vi "1-Tap 8-bit Camera with Bayer (Host).vi"() -> ()   [LabVIEW 2012]
doc: "This is the host VI for the 1-Tap 8-Bit Camera with Bayer example. This example demonstrates how to acquire images from a 1-tap, 8-bit, base configuration, Camera Link camera with a color sensor and display the images on the host.\n\nThis example also demonstrates the use of third-party IP imported into the LabVIEW project as a CLIP. In this case, the imported CLIP comes from an FPGA netlist and performs the Bayer color decoding to convert the incoming 8-bit Bayer images into 24-bit RGB images in real time.\n\nAdditionally, the example demonstrates the serial server, which allows third-party camera configuration utilities to communicate with the camera using the Camera Link serial interface while this VI is running."
uses:
  <vilib>/userdefined/High Color/nirio_resource_hc.ctl
  <vilib>/FPGAPlugInAG/PCIe-1473R/niLvFpga_Open_PCIe-1473R.vi
  <vilib>/rvi/interface/common/dynamic/niFpgaDynamicAddResources.vi
  <vilib>/FPGAPlugInAG/Dynamic/niLvFpga_Reset_Dynamic.vi
  <vilib>/Utility/error.llb/Error Cluster From Error Code.vi
  <vilib>/rvi/errors/niLvFpgaAdjustHostInterfaceError.vi
  <vilib>/FPGAPlugInAG/Dynamic/niLvFpga_Run_Dynamic.vi
  <vilib>/FPGAPlugInAG/Dynamic/niLvFpga_Close_Dynamic.vi
  <vilib>/rvi/interface/nirviOpenFPGA/nirviOpenFPGA.xnode
  FPGA Bitfiles/1-Tap8-bitCamera_FPGATarget_1-Tap8-bitCamera_6EA2B931.lvbitx
  1-Tap 8-Bit Camera with Bayer (FPGA).vi
  <vilib>/rvi/interface/nirviMethod/nirviMethod.xnode
  <vilib>/rvi/interface/nirviReadWriteControl/nirviReadWriteControl.xnode
  <vilib>/rvi/interface/nirviCloseFPGA/nirviCloseFPGA.xnode
  NiFpgaLv.dll
  <vilib>/rvi/interface/Simulation/niFpgaSimulationCallBeginRW.vi
  <vilib>/rvi/errors/niLvFpgaMergeErrorWithErrorCode.vi
  <vilib>/FPGAPlugInAG/Dynamic/niLvFpga_ConfigureFifo_Dynamic.vi
  <vilib>/FPGAPlugInAG/Dynamic/niLvFpga_StartFifo_Dynamic.vi
  <vilib>/FPGAPlugInAG/Dynamic/niLvFpga_ReadFifo_Dynamic.vi
panel:
  in  "Bayer Pattern":u16(ring) items=["GBGB::RGRG", "GRGR::BGBG", "BGBG::GRGR", "RGRG::GBGB"]
  out "Acq In Progress":bool
  in  "Frames To Acquire":u32=1 caption="Frames To Acquire\n(0 = infinite)"
  in  "Cancel":bool
  out "Acq'd Frame Width":u32
  in  "Stopped":bool
  in  "RIO Device":T1="RIO0"
  out "DMA Write Timeout":bool
  in  "Start Serial Server":bool=TRUE
  out "Frames Acq'd":u32
  out "Acq'd Frame Height":u32
  out "Image":T2(plugin-control)
  in  "Acquire":bool
  in  "Stop":bool
  in  "Image Height":u32=480 max=65535
  in  "Image Width":u32=640 max=65535
  out "Initialized":bool
  # "Note: The decoded output image is two columns\nand two rows smaller than the input image."
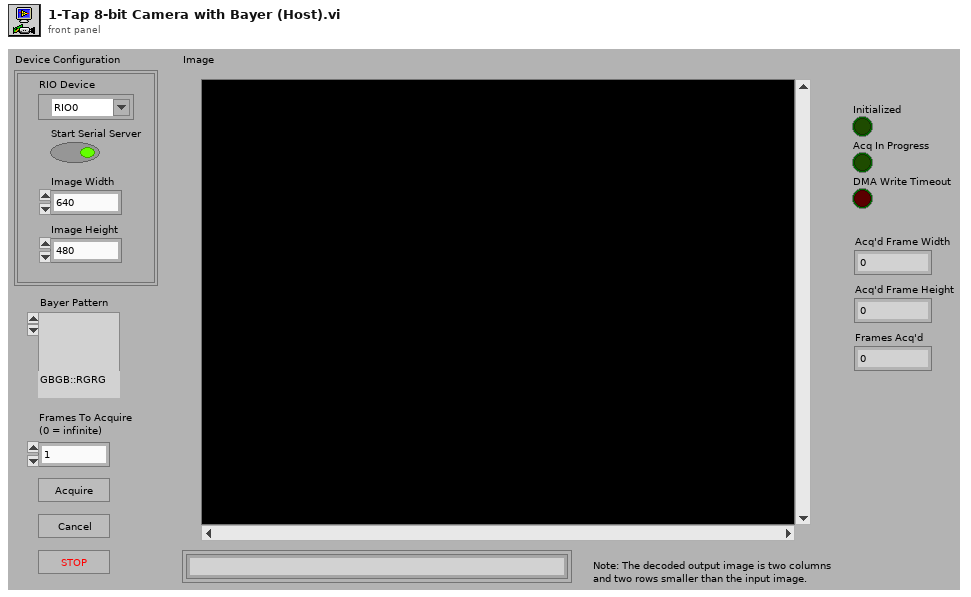
[diagram p1: front panel]
types:
  T1 = typedef "nirio_resource_hc.ctl" = tag
  T2 = typedef "IMAQ Image.ctl" = refnum<image>
  T3 = enum8{"Standard", "Basler 10-tap", "Vosskühler 10-tap"}
  T4 = typedef "Image Type" = u32
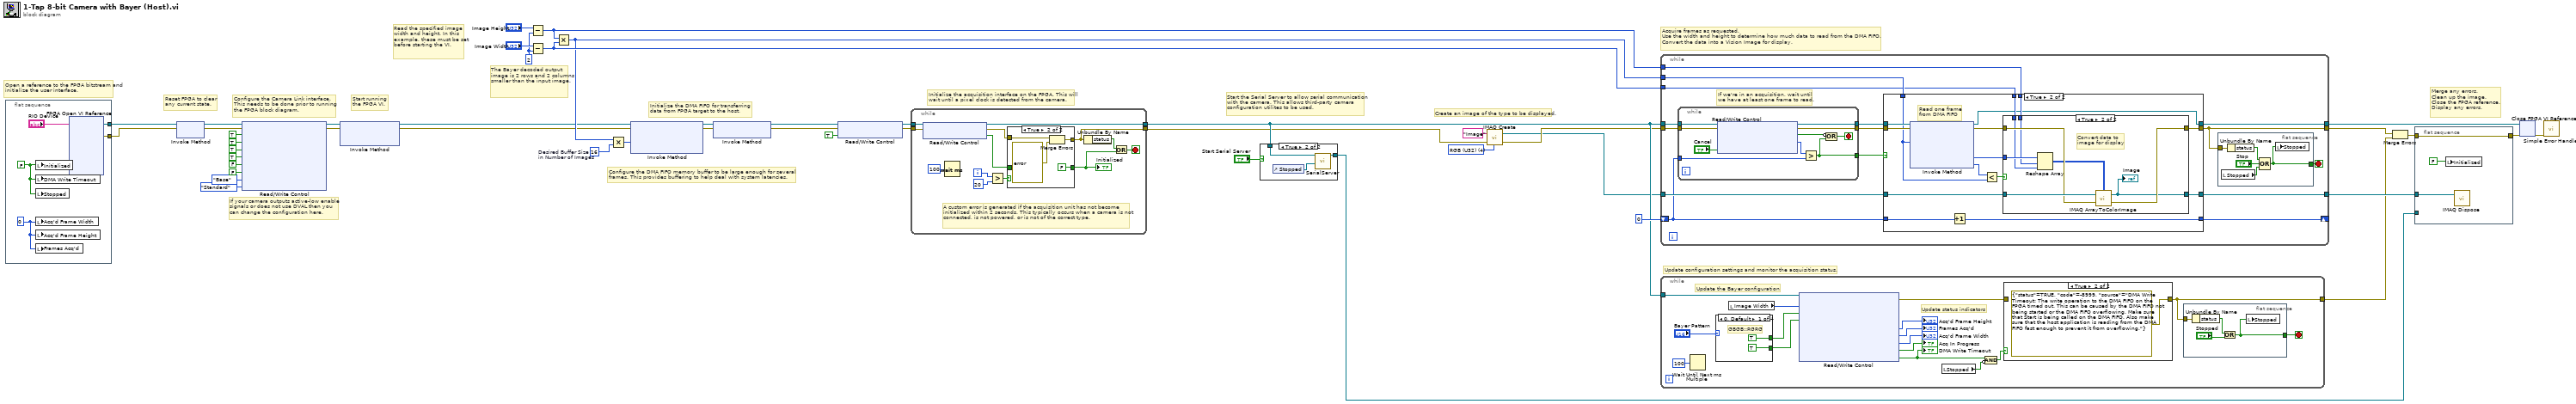
[diagram p0: block diagram]
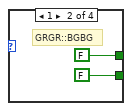
[diagram p3: hidden frame]
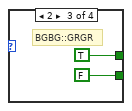
[diagram p4: hidden frame]
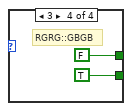
[diagram p5: hidden frame]
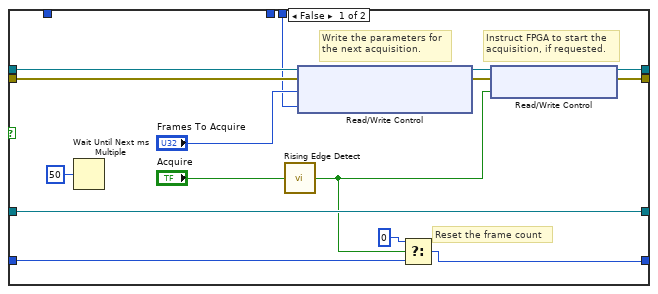
[diagram p7: hidden frame]
diagram:
  w6 = u32 2 ("y")
  w43 = T4 4 items=["Grayscale (U8)", "Grayscale (I16)", "Grayscale (SGL)", "Complex (CSG)", "RGB (U32)", "HSL (U32)", "RGB (U64)", "Grayscale (U16)"] ("Image Type")
  w17 = u32 16  # Desired Buffer Size in Number of Images
  # "The Bayer decoded output image is 2 rows and 2 columns smaller than the input image."
  # "If your camera outputs active-low enable\nsignals or does not use DVAL then you\ncan change the configuration here."
  # "Configure the DMA FIFO memory buffer to be large enough for several\nframes. This provides buffering to help deal with system latencies."
  # "Start running\nthe FPGA VI."
  # "Reset FPGA to clear\nany current state."
  # "Read the specified image width and height. In this example, these must be set before starting the VI."
  # "Merge any errors.\nClean up the image.\nClose the FPGA reference.\nDisplay any errors."
  # "Acquire frames as requested.\nUse the width and height to determine how much data to read from the DMA FIFO.\nConvert the data into a Vision Image for display."
  # "Update configuration settings and monitor the acquisition status."
  # "Start the Serial Server to allow serial communication\nwith the camera. This allows third-party camera\nconfiguration utilites to be used."
  # "Create an image of the type to be displayed."
  # "Initialize the acquisition interface on the FPGA. This will\nwait until a pixel clock is detected from the camera."
  # "Initialize the DMA FIFO for transferring\ndata from FPGA target to the host."
  # "Configure the Camera Link interface.\nThis needs to be done prior to running\nthe FPGA block diagram."
  # "Open a reference to the FPGA bitstream and initialize the user interface."
  n1 = flat-sequence {
    tunnel: [w49] -> w36
    tunnel: [w48] -> w47
    frame #0 {
      w52 = u32 0 ("Num Lines Acq'd")
      w51 = FALSE ("stop")
      n2 = local write "Initialized"(w51) -> ()
      n3 = local write "DMA Write Timeout"(w51) -> ()
      n4 = local write "Stopped"(w51) -> ()
      n5 = local write "Acq'd Frame Width"(w52) -> ()
      n6 = local write "Acq'd Frame Height"(w52) -> ()
      n7 = local write "Frames Acq'd"(w52) -> ()
      n8 = xnode "FPGA Open VI Reference"("resource name"="RIO Device") -> ("FPGA VI Reference Out"=w49:refnum<k20>, "error out"=w48:errorcluster)  [unwired: 1 in]
    }
  }
  n9 = xnode "Invoke Method"("FPGA VI Reference In"=w36, "error in"=w47) -> ("FPGA VI Reference Out"=w25:refnum<k20>, "error out"=w28:errorcluster)
  n10 = xnode "Read/Write Control"("FPGA VI Reference In"=w25, "error in"=w28, "CL Config.FVAL Active High"=TRUE ("IO Module Config.CL FVAL Active High"), "CL Config.LVAL Active High"=TRUE ("IO Module Config.CL LVAL Active High"), "CL Config.DVAL Active High"=TRUE ("IO Module Config.CL DVAL Active High"), "CL Config.Spare Active High"=TRUE ("IO Module Config.CL Spare Active High"), "CL Config.Line Scan"=FALSE ("Line Scan"), "Acq Control.Ignore DVAL"=FALSE ("CL Config.Line Scan"), "CL Config.Configuration"=enum8{"Base", "Medium", "Full"}."Base", "CL Config.Signal Mapping"=T3."Standard") -> ("FPGA VI Reference Out"=w29:refnum<k20>, "error out"=w27:errorcluster)
  n11 = xnode "Invoke Method"("FPGA VI Reference In"=w29, "error in"=w27) -> ("FPGA VI Reference Out"=w2:refnum<k20>, "error out"=w1:errorcluster)  [unwired: 1 in]
  n12 = Subtract(x="Image Height", y=w6) -> (x-y=w8:u32)
  n13 = Subtract(x="Image Width", y=w6) -> (x-y=w7:u32)
  n14 = Multiply(x=w8, y=w7) -> (x*y=w5:u32)
  n15 = Multiply(x=w5, y=w17) -> (x*y=w19:u32)
  n16 = xnode "Invoke Method"("FPGA VI Reference In"=w2, "error in"=w1, "Requested Depth"=w19) -> ("FPGA VI Reference Out"=w35:refnum<k20>, "error out"=w34:errorcluster)  [unwired: 1 out]
  n17 = xnode "Invoke Method"("FPGA VI Reference In"=w35, "error in"=w34) -> ("FPGA VI Reference Out"=w20:refnum<k20>, "error out"=w33:errorcluster)
  n18 = xnode "Read/Write Control"("FPGA VI Reference In"=w20, "error in"=w33, "Acq Control.Initialize"=TRUE ("Arm Acquisition")) -> ("FPGA VI Reference Out"=w46:refnum<k20>, "error out"=w45:errorcluster)
  n19 = while {
    tunnel: w46 -> [w60]
    tunnel: w45 -> [w59]
    tunnel: [w58] -> w16
    tunnel: [w62] -> w15
    i -> [w54]
    stop <- w65 stop-if-true
    # "A custom error is generated if the acquisition unit has not become initialized within 2 seconds. This typically occurs when a camera is not connected, is not powered, or is not of the correct type."
    n20 = xnode "Read/Write Control"("FPGA VI Reference In"=w60, "error in"=w59) -> ("FPGA VI Reference Out"=w58:refnum<k20>, "error out"=w57:errorcluster, "Acq Status.Initialized"=w56:bool)
    n21 = Wait (ms)(milliseconds to wait=u32 100) -> ()  [unwired: 1 out]
    n22 = Greater?(x=w54, y=20) -> (0:w55:bool)
    n23 = case shown="True" w55 {
      tunnel: [w67 FALSE] -> w61
      tunnel: w56 -> [w67 _]
      tunnel: w57 -> [w66 w69]
      tunnel: [w66 w71] -> w62
      frame False {
      }
      frame True {
        n24 = Merge Errors(w69, errorcluster {"status"=TRUE, "code"=-8999, "source"="Acquisition Initialization: This error typically occurs when a camera is not properly connected, is not powered, or is not of the correct type."} ("error in")) -> (w71:errorcluster)
      }
    }
    "Initialized" <- w61
    n25 = Unbundle By Name(w62) -> ("status"=w64:bool)
    n26 = Or(x=w64, y=w61) -> (x .or. y?=w65:bool)
  }
  n27 = case shown="True" "Start Serial Server" {
    tunnel: [_ w72] -> w37
    tunnel: w16 -> [_ w73]
    frame False {
    }
    frame True {
      n28 = control-ref of="Stopped"() -> (w74:refnum<vi>)
      n29 = call "SerialServer.vi"("Stop Refnum"=w74, "FPGA VI Reference In"=w73) -> ("FPGA VI Reference Out"=w72:refnum<k20>)  [unwired: 5 in]
    }
  }
  n30 = call "IMAQ Create"("Image Name"="Image", "Image Type"=w43, "error in (no error)"=w15) -> ("New Image"=w11:T2, "error out"=w12:errorcluster)  [unwired: 2 in]
  n31 = while {
    tunnel: w16 -> [w81]
    tunnel: w12 -> [w80]
    tunnel: w5 -> [w89]
    tunnel: w8 -> [w88]
    tunnel: w7 -> [w87]
    tunnel: w11 -> [w86]
    tunnel: [w84] -> w31
    tunnel: [w85] -> w42
    tunnel: [w82] -> w39
    shift-right: [w76] -> _
    shift-left: u32 0 -> [w75]
    stop <- w83 stop-if-true
    # "If we're in an acquisition, wait until \nwe have at least one frame to read."
    n32 = while {
      tunnel: w81 -> [w96]
      tunnel: w80 -> [w95]
      tunnel: [w93] -> w79
      tunnel: [w94] -> w78
      tunnel: w75 -> [w99]
      tunnel: [w97] -> w77
      stop <- w98 stop-if-true
      n33 = xnode "Read/Write Control"("FPGA VI Reference In"=w96, "error in"=w95, "Acq Control.Cancel Acq"="Cancel") -> ("FPGA VI Reference Out"=w94:refnum<k20>, "error out"=w93:errorcluster, "Acq Status.Acq In Progress"=w92:bool, "Acq Status.Frames Acq'd"=w91:u32)
      n34 = Greater?(x=w91, y=w99) -> (0:w97:bool)
      n35 = Compound Arithmetic op=OR(invert w92, w97) -> (w98:bool)
    }
    n36 = case shown="True" w77 {
      tunnel: w78 -> [w115 w130]
      tunnel: w79 -> [w114 w129]
      tunnel: w89 -> [_ w122]
      tunnel: w88 -> [w112 w124]
      tunnel: w87 -> [_ w125]
      tunnel: w86 -> [w119 w134]
      tunnel: [w108 w132] -> w84
      tunnel: [w111 w120] -> w85
      tunnel: [w119 w131] -> w82
      tunnel: w75 -> [w116 w128]
      tunnel: [w118 w127] -> w76
      frame False {
        # "Reset the frame count"
        # "Instruct FPGA to start the\nacquisition, if requested."
        # "Write the parameters for\nthe next acquisition."
        n37 = Wait Until Next ms Multiple(millisecond multiple=u32 50) -> ()  [unwired: 1 out]
        n38 = call "Rising Edge Detect.vi"("Input"="Acquire") -> ("Pulse"=w105:bool)  [unwired: 4 in]
        n39 = xnode "Read/Write Control"("FPGA VI Reference In"=w115, "error in"=w114, "Acq Control.Frames To Acq"="Frames To Acquire", "Acq Control.Line Scan Height"=w112) -> ("FPGA VI Reference Out"=w110:refnum<k20>, "error out"=w109:errorcluster)
        n40 = Select(t=u32 0, s=w105, f=w116) -> (s? t:f=w118:u32)
        n41 = xnode "Read/Write Control"("FPGA VI Reference In"=w110, "error in"=w109, "Acq Control.Acquire"=w105) -> ("FPGA VI Reference Out"=w111:refnum<k20>, "error out"=w108:errorcluster)
      }
      frame True {
        # "Read one frame\nfrom DMA FIFO"
        n42 = xnode "Invoke Method"("FPGA VI Reference In"=w130, "error in"=w129, "Number of Elements"=w122) -> ("FPGA VI Reference Out"=w120:refnum<k20>, "error out"=w133:errorcluster, "Data"=w126:u32[], "Elements Remaining"=w123:u32)  [unwired: 1 in]
        n43 = Increment(x=w128) -> (x+1=w127:u32)
        n44 = Less?(x=w123, y=w122) -> (x < y?=w121:bool)
        n45 = case shown="True" w121 {
          tunnel: w134 -> [w136 w144]
          tunnel: w133 -> [w135 w143]
          tunnel: [w135 w142] -> w132
          tunnel: [w136 w141] -> w131
          tunnel: w126 -> [_ w140]
          tunnel: w125 -> [_ w138]
          tunnel: w124 -> [_ w137]
          frame False {
            # "Do not display the image if we're\nfalling behind in the acquisition."
          }
          frame True {
            # "Convert data to\nimage for display"
            n46 = Reshape Array(w140, w137, w138) -> (w139:u32[][])
            n47 = call "IMAQ ArrayToColorImage"("Image Pixels (U32)"=w139, "Image"=w144, "error in (no error)"=w143) -> ("Image Out"=w141:T2, "error out"=w142:errorcluster)  [unwired: 2 in]
            "Image" <- w141
          }
        }
      }
    }
    n48 = flat-sequence {
      tunnel: w84 -> [w102]
      tunnel: [w101] -> w83
      frame #0 {
        n49 = local read "Stopped"() -> (w100:bool)
        n50 = Unbundle By Name(w102) -> ("status"=w103:bool)
        n51 = Compound Arithmetic op=OR(w103, "Stop", w100) -> (w101:bool)
        n52 = local write "Stopped"(w101) -> ()
      }
    }
  }
  n53 = while {
    tunnel: w16 -> [w157]
    tunnel: [w160] -> w30
    stop <- w159 stop-if-true
    # "Update the Bayer configuration"
    # "Update status indicators"
    n54 = Wait Until Next ms Multiple(millisecond multiple=u32 100) -> ()  [unwired: 1 out]
    n55 = case shown="0, Default" "Bayer Pattern" {
      tunnel: [TRUE FALSE TRUE FALSE] -> w149
      tunnel: [TRUE FALSE FALSE TRUE] -> w148
      frame 0, Default {
        # "GBGB::RGRG"
      }
      frame 1 {
        # "GRGR::BGBG"
      }
      frame 2 {
        # "BGBG::GRGR"
      }
      frame 3 {
        # "RGRG::GBGB"
      }
    }
    n56 = local read "Image Width"() -> (w150:u32)
    n57 = xnode "Read/Write Control"("FPGA VI Reference In"=w157, "Bayer Decoder.Image Width"=w150, "Bayer Decoder.First Row Is Blue"=w149, "Bayer Decoder.First Column Is Red"=w148) -> ("error out"=w156:errorcluster, "Acq Status.Lines Per Frame"=→"Acq'd Frame Height":u32, "Acq Status.Frames Acq'd"=→"Frames Acq'd":u32, "Acq Status.Clocks Per Line"=→"Acq'd Frame Width":u32, "Acq Status.Acq In Progress"=→"Acq In Progress":bool, "Acq Status.DMA Write Timeout"=w145:bool)  [unwired: 1 in, 1 out]
    "DMA Write Timeout" <- w145
    n58 = local read "Stopped"() -> (w146:bool)
    n59 = Compound Arithmetic op=AND(w145, invert w146) -> (w147:bool)
    n60 = case shown="True" w147 {
      tunnel: w156 -> [w173 _]
      tunnel: [w173 errorcluster {"status"=TRUE, "code"=-8999, "source"="DMA Write Timeout: The write operation to the DMA FIFO on the FPGA timed out. This can be caused by the DMA FIFO not being started or the DMA FIFO overflowing. Make sure that Start is being called on the DMA FIFO. Also make sure that the host application is reading from the DMA FIFO fast enough to prevent it from overflowing."} ("error out")] -> w160
      frame False {
      }
      frame True {
      }
    }
    n61 = flat-sequence {
      tunnel: w160 -> [w172]
      tunnel: [w170] -> w159
      frame #0 {
        n62 = Unbundle By Name(w172) -> ("status"=w171:bool)
        n63 = Or(x=w171, y="Stopped") -> (x .or. y?=w170:bool)
        n64 = local write "Stopped"(w170) -> ()
      }
    }
  }
  n65 = Merge Errors(w31, w30) -> (w32:errorcluster)
  n66 = flat-sequence {
    tunnel: w32 -> [w176]
    tunnel: [w176] -> w41
    tunnel: w39 -> [w177]
    tunnel: w37 -> [_]
    frame #0 {
      n67 = local write "Initialized"(FALSE ("Module Enabled")) -> ()
      n68 = call "IMAQ Dispose"("Image"=w177) -> ()  [unwired: 5 in, 1 out]
    }
  }
  n69 = xnode "Close FPGA VI Reference"("FPGA VI Reference In"=w42, "error in"=w41) -> ("error out"=w38:errorcluster)
  n70 = call <vilib>:"Simple Error Handler.vi"("error in (no error)"=w38) -> ()  [unwired: 4 in, 5 out]
